vi "Features_SpecPage.vi"(10 "Spec Page Interface":T1, 11 "MetaDataObj in":refnum<class "MetaDataObj.lvclass">) -> (3 "MetaDataObj out":refnum<class "MetaDataObj.lvclass">)   [LabVIEW 2013, in "editorscriptingobject.lvclass"]
uses:
  editorscriptingobject.lvclass
  <resource>/dialog/NewProjectWizard/Spec Page Interface.ctl
  <resource>/dialog/NewProjectWizard/MetaDataObj/MetaDataObj.lvclass
  <resource>/dialog/NewProjectWizard/MetaDataObj/MetaDataObj.lvclass/MetaDataObj.ctl
  editorscriptingobject.lvclass/editorscriptingobject.ctl
  <resource>/dialog/NewProjectWizard/MetaDataObj/Accessors/Write Project Name.vi
  <resource>/dialog/NewProjectWizard/MetaDataObj/Accessors/Write Project Root.vi
  Write library name.vi
  <resource>/dialog/NewProjectWizard/MetaDataObj/Accessors/Write File Prefix.vi
panel:
  in  "Configuration *.lvlib File Name":string
  in  "Project Name":string
  in  "Project Root":path
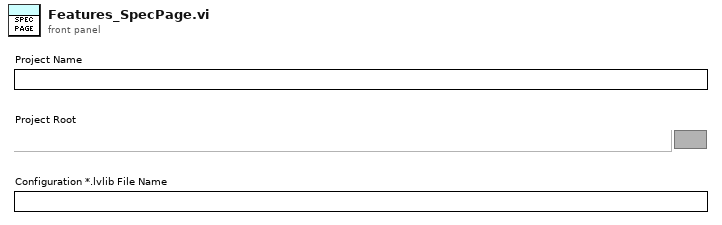
[diagram p1: front panel]
types:
  T1 = typedef "Spec Page Interface.ctl" = cluster{"\"Tab Forward To\" Refnum":refnum<vi>, "\"Tab Backward To\" Refnum":refnum<vi>, "Errors":refnum<user-event>, "Quit":refnum<user-event>}
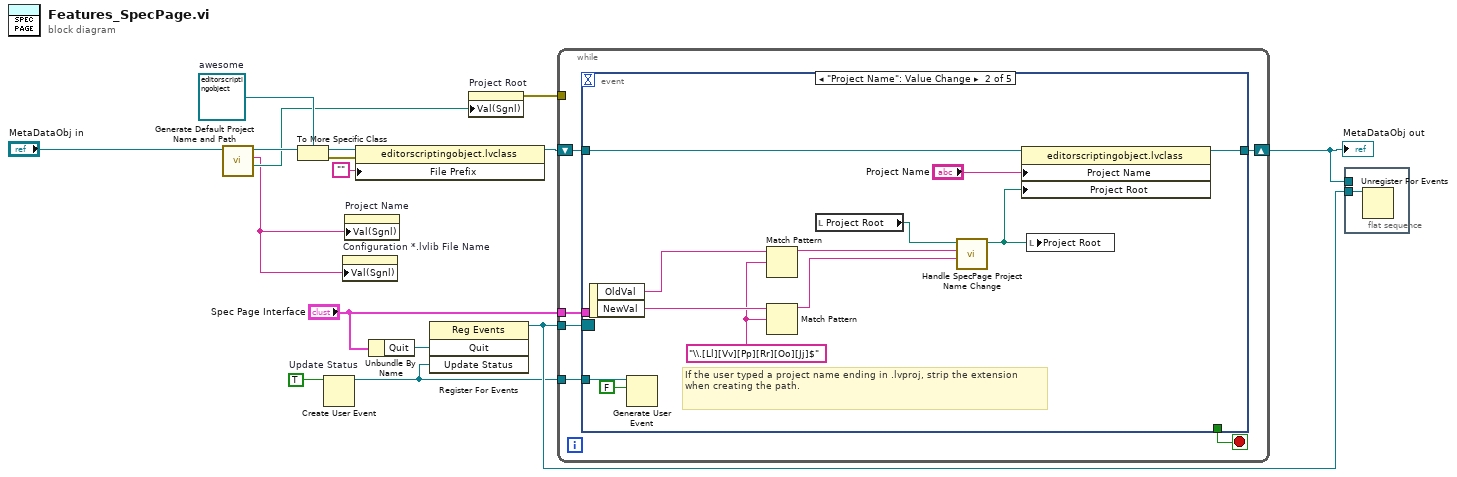
[diagram p0: block diagram]
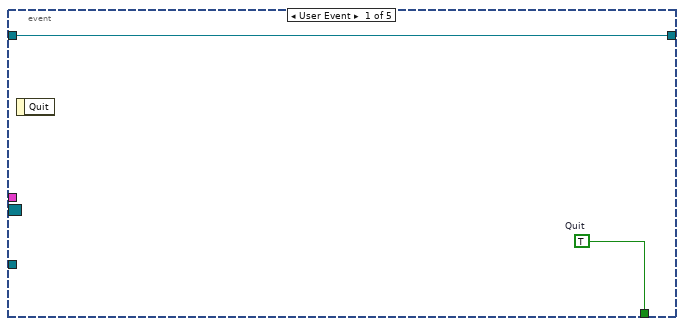
[diagram p2: hidden frame]
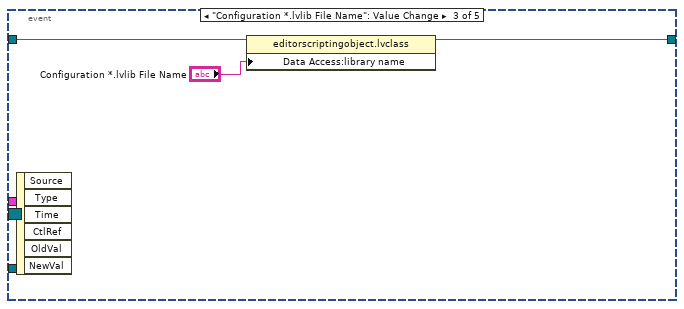
[diagram p3: hidden frame]
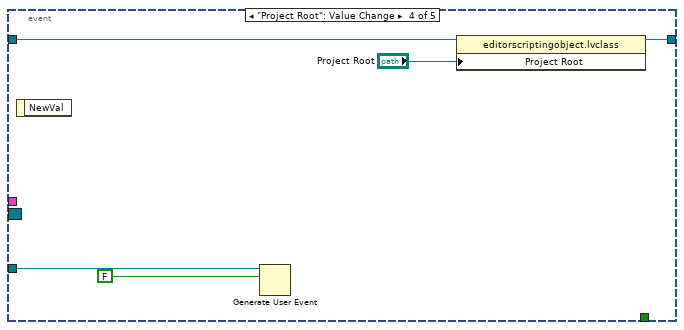
[diagram p4: hidden frame]
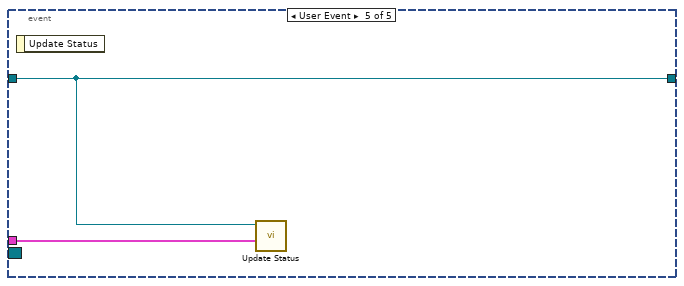
[diagram p5: hidden frame]
diagram:
  w10 = TRUE  # Update Status
  w11 = refnum<class "editorscriptingobject.lvclass"> refnum  # awesome
  n1 = call <resource>:"Generate Default Project Name and Path.vi"("DNL_MetaDataObj in"="MetaDataObj in") -> ("Project Root"=w3:path, "Project Name"=w1:string, "DNL_MetaDataObj out"=w4:refnum<class "MetaDataObj.lvclass">)  [unwired: 8 in]
  n2 = To More Specific Class(target class=w11, reference=w4) -> (specific class reference=w13:refnum<class "editorscriptingobject.lvclass">, error out=w12:errorcluster)  [unwired: 1 in]
  n3 = Create User Event(user event datatype=w10) -> (user event=w7:refnum<user-event>)  [unwired: 1 in, 1 out]
  n4 = property on="Configuration *.lvlib File Name" class="Str"("Val(Sgnl)"=w1) -> ()  [unwired: 2 in, 2 out]
  n5 = property on="Project Name" class="Str"("Val(Sgnl)"=w1) -> ()  [unwired: 2 in, 2 out]
  n6 = property class="editorscriptingobject.lvclass"(reference=w13, error in=w12, "File Prefix"="") -> (reference out=w9:refnum<class "editorscriptingobject.lvclass">)  [unwired: 1 out]
  n7 = Unbundle By Name("Spec Page Interface") -> ("Quit"=w16:refnum<user-event>)
  n8 = register-events(w16, w7) -> (reference out=w15:refnum<event-registration>)  [unwired: 2 in, 1 out]
  n9 = property on="Project Root" class="Path"("Val(Sgnl)"=w3) -> (error out=w8:errorcluster)  [unwired: 2 in, 1 out]
  n10 = while {
    tunnel: "Spec Page Interface" -> [w21]
    shift-right: [w19] -> w2
    shift-left: w9 -> [w18]
    tunnel: w15 -> [w20]
    tunnel: w8 -> [_]
    tunnel: w7 -> [w17]
    stop <- w22 stop-if-true
    n11 = event shown="[1] \"Project Name\": Value Change" {
      selector: w20 -> [_ _ _ _ _]
      dyn-events: _ -> [_ _ _ _ _]
      timeout: _ -> [_ _ _ _ _]
      tunnel: w21 -> [_ _ _ _ w45]
      tunnel: [w24 _ _ _ _] -> w22
      tunnel: [w23 w36 w38 w43 w46] -> w19
      tunnel: w18 -> [w23 w33 w39 w44 w46]
      tunnel: w17 -> [_ w35 _ w42 _]
      event User Event {
        w24 = TRUE  # Quit
        n12 = event-data() -> ()  [unwired: 1 in, 1 out]
      }
      event "Project Name": Value Change {
        w28 = "\\.[Ll][Vv][Pp][Rr][Oo][Jj]$" ("regular expression")
        # "If the user typed a project name ending in .lvproj, strip the extension when creating the path."
        n13 = event-data() -> ("OldVal"=w30:string, "NewVal"=w29:string)  [unwired: 1 in]
        n14 = Generate User Event(user event=w35, event data cluster=FALSE ("Update Status")) -> ()  [unwired: 2 in, 2 out]
        n15 = Match Pattern(string=w30, regular expression=w28) -> (before substring=w27:string)  [unwired: 1 in, 3 out]
        n16 = Match Pattern(string=w29, regular expression=w28) -> (before substring=w26:string)  [unwired: 1 in, 3 out]
        n17 = local read "Project Root"() -> (w32:path)
        n18 = call <resource>:"Handle SpecPage Project Name Change.vi"("Project Name New Value"=w26, "Project Name Old Value"=w27, "Project Root in"=w32) -> ("Project Root out"=w31:path)  [unwired: 8 in]
        n19 = property class="editorscriptingobject.lvclass"(reference=w33, "Project Name"="Project Name", "Project Root"=w31) -> (reference out=w36:refnum<class "editorscriptingobject.lvclass">)  [unwired: 1 in, 1 out]
        n20 = local write "Project Root"(w31) -> ()
      }
      event "Configuration *.lvlib File Name": Value Change {
        n21 = event-data() -> ()  [unwired: 1 in, 6 out]
        n22 = property class="editorscriptingobject.lvclass"(reference=w39, "Data Access:library name"="Configuration *.lvlib File Name") -> (reference out=w38:refnum<class "editorscriptingobject.lvclass">)  [unwired: 1 in, 1 out]
      }
      event "Project Root": Value Change {
        n23 = event-data() -> ()  [unwired: 1 in, 1 out]
        n24 = Generate User Event(user event=w42, event data cluster=FALSE ("Update Status")) -> ()  [unwired: 2 in, 2 out]
        n25 = property class="editorscriptingobject.lvclass"(reference=w44, "Project Root"="Project Root") -> (reference out=w43:refnum<class "editorscriptingobject.lvclass">)  [unwired: 1 in, 1 out]
      }
      event User Event {
        n26 = event-data() -> ()  [unwired: 1 in, 1 out]
        n27 = call "Update Status.vi"("Spec Page Interface"=w45, "TwoTasksMetaDataObj in"=w46) -> ()  [unwired: 10 in]
      }
    }
  }
  "MetaDataObj out" <- w2
  n28 = flat-sequence {
    tunnel: w15 -> [w47]
    tunnel: w2 -> [_]
    frame #0 {
      n29 = Unregister For Events(event registration refnum=w47) -> ()  [unwired: 1 in, 1 out]
    }
  }
